vi "Editor UI.vi"(10 "Close Event":refnum<user-event>, 11 "Simulated PSU in":refnum<class "Simulated PSU.lvclass">) -> ()   [LabVIEW 2020, in "Simulated PSU.lvlib" / "Simulated PSU.lvclass"]
uses:
  Simulated PSU.lvclass
  build/ppl/lv-hal.lvlibp/Device/Editor Event Data.ctl
  Simulated PSU.lvclass/Simulated PSU.ctl
  build/ppl/lv-hal.lvlibp/Device/Device.lvclass
  C:/dev/HAL Demo/build/ppl/lv-hal.lvlibp/Device/Device.lvclass
panel:
  in  "Noise Factor (0-1)":dbl min=0.0 max=1.0 format="%#_6f"
  in  "Simulated\nResistance":dbl format="%#_6f Ohms"
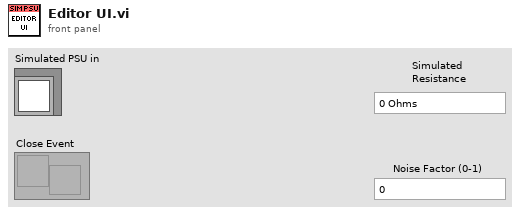
[diagram p1: front panel]
types:
  T1 = typedef "Simulated PSU.lvlib/Simulated PSU.lvclass/Ref Data.ctl" = cluster{"Enabled":bool, "Voltage":dbl, "Noise Level":dbl, "Resistance":dbl}
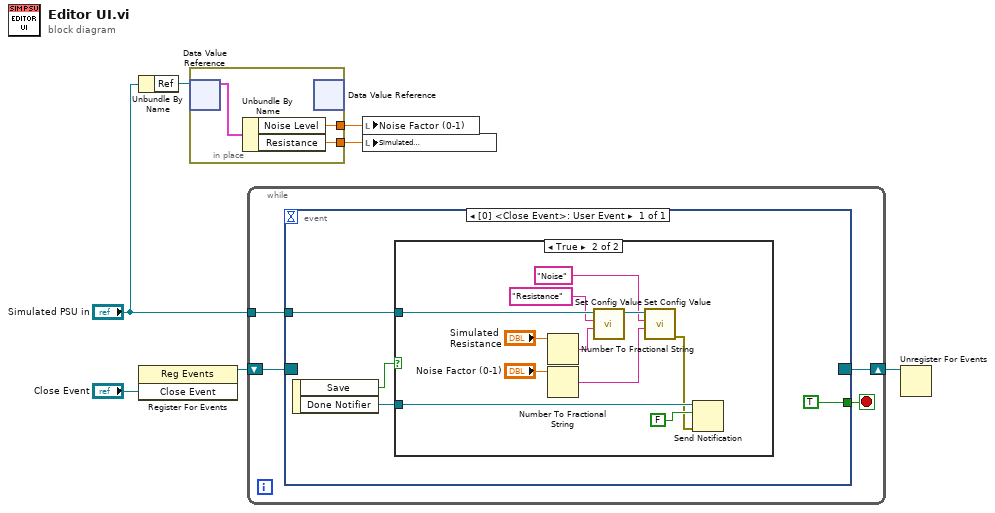
[diagram p0: block diagram]
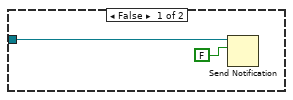
[diagram p2: hidden frame]
diagram:
  n1 = Unbundle By Name("Simulated PSU in") -> ("Ref"=w4:refnum<data-value>)
  n2 = register-events("Close Event") -> (reference out=w6:refnum<event-registration>)  [unwired: 2 in, 1 out]
  n3 = in-place {
    in-place-border: [w9] -> w1
    in-place-border: [w8] -> w2
    n4 = in-place-dvr #1(w4) -> (w10:T1)  [unwired: 1 out]
    n5 = Unbundle By Name(w10) -> ("Noise Level"=w9:dbl, "Resistance"=w8:dbl)
    n6 = in-place-dvr #1() -> ()  [unwired: 1 in, 2 out]
  }
  n7 = while {
    shift-right: [w12] -> w5
    shift-left: w6 -> [w14]
    tunnel: "Simulated PSU in" -> [w13]
    stop <- w11 stop-if-true
    n8 = event shown="[0] <Close Event>: User Event" {
      selector: w14 -> [_]
      dyn-events: [_] -> w12
      timeout: _ -> [_]
      tunnel: w13 -> [w17]
      tunnel: [TRUE] -> w11
      event User Event {
        n9 = event-data() -> ("Save"=w18:bool, "Done Notifier"=w15:refnum<notifier>)  [unwired: 1 in]
        n10 = case shown="True" w18 {
          tunnel: w17 -> [_ w31]
          tunnel: w15 -> [w20 w22]
          frame False {
            n11 = Send Notification(notification=FALSE, notifier=w20) -> ()  [unwired: 1 in, 2 out]
          }
          frame True {
            n12 = Number To Fractional String(number="Simulated\nResistance") -> (F-format string=w27:string)  [unwired: 3 in]
            n13 = Number To Fractional String(number="Noise Factor (0-1)") -> (F-format string=w26:string)  [unwired: 3 in]
            n14 = call "Set Config Value.vi"("Value"=w27, "Config Key"="Resistance", "Device in"=w31) -> ("Device out"=w30:refnum<class "Simulated PSU.lvclass">)  [unwired: 7 in, 1 out]
            n15 = call "Set Config Value.vi"("Value"=w26, "Config Key"="Noise", "Device in"=w30) -> ("error out"=w21:errorcluster)  [unwired: 7 in, 1 out]
            n16 = Send Notification(notification=FALSE, notifier=w22, error in (no error)=w21) -> ()  [unwired: 2 out]
          }
        }
      }
    }
  }
  n17 = local write "Noise Factor (0-1)"(w1) -> ()
  n18 = local write "Simulated\nResistance"(w2) -> ()
  n19 = Unregister For Events(event registration refnum=w5) -> ()  [unwired: 1 in, 1 out]
